vi "Required Buffer Size.vi"(8 "error in (no error)":errorcluster, 11 "Transfer Group Configuration in":refnum<class "Transfer Group Configuration.lvclass">) -> (0 "error out":errorcluster, 2 "required buffer size":u64 format="%d bytes", 3 "Transfer Group Configuration out":refnum<class "Transfer Group Configuration.lvclass">)   [LabVIEW 2017, in "DSF Core.lvlib" / "Transfer Group Configuration.lvclass"]
uses:
  Transfer Group Configuration.lvclass
  Transfer Group Configuration.lvclass/Transfer Group Configuration.ctl
  Transfer/Transfer Configuration.lvclass
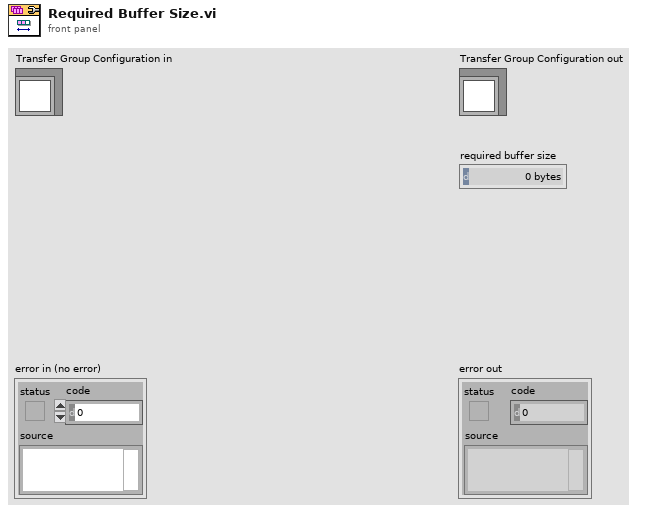
[diagram p1: front panel]
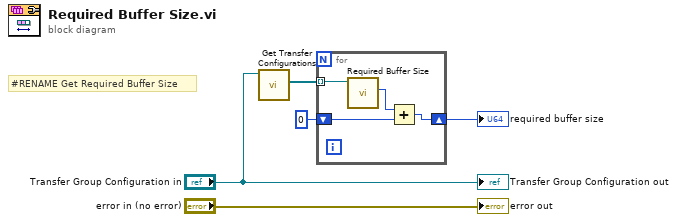
[diagram p0: block diagram]
diagram:
  # "#RENAME Get Required Buffer Size"
  n1 = call "Get Transfer Configurations.vi"("Transfer Group Configuration in"="Transfer Group Configuration in") -> ("Transfer Configurations"=w3:refnum<class "Transfer Configuration.lvclass">[])  [unwired: 9 in, 1 out]
  n2 = for {
    tunnel: w3 -> [w6] mode=indexing
    shift-right: [w8] -> w1
    shift-left: u64 0 -> [w7]
    n3 = call "Required Buffer Size.vi"("Transfer Configuration in"=w6) -> ("required buffer size"=w9:u64)  [unwired: 8 in, 2 out]
    n4 = Add(x=w9, y=w7) -> (x+y=w8:u64)
  }
  "required buffer size" <- w1
  "error out" <- "error in (no error)"
  "Transfer Group Configuration out" <- "Transfer Group Configuration in"
